vi "testStringNotIncluded.vi"(9 "haystack":string, 10 "needle":string) -> (0 "error out":errorcluster)   [LabVIEW 2019, in "AssertionTest.lvlib" / "AssertStringContainsString.lvlib"]
uses:
  AssertStringContainsString.lvlib
  Assertion/Assertion.lvlib
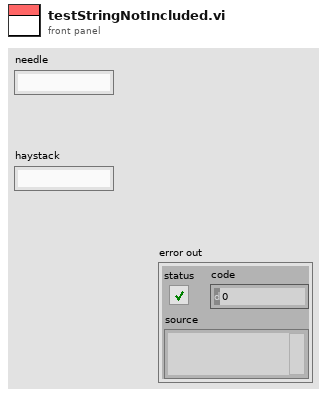
[diagram p1: front panel]
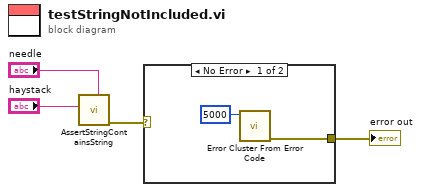
[diagram p0: block diagram]
diagram:
  n1 = call "AssertStringContainsString.vi"("Needle"="needle", "Haystack"="haystack") -> ("error out"=w4:errorcluster)  [unwired: 9 in]
  n2 = case shown="No Error" w4 {
    tunnel: [w5 _] -> w1
    frame No Error {
      n3 = call <vilib>:"Error Cluster From Error Code.vi"("error code (0)"=5000) -> ("error out"=w5:errorcluster)  [unwired: 8 in]
    }
    frame Error {
    }
  }
  "error out" <- w1
